vi "leitura de serial.vi"() -> ()   [LabVIEW 2025]
uses:
  <vilib>/Instr/_visa.llb/VISA Configure Serial Port (Instr).vi
panel:
  out "Waveform Chart 2":dbl(graph)
  out "output 2":dbl
  out "Waveform Chart":dbl(graph)
  out "output 1":dbl
  in  "termination char\n(0xA = '\\n' = LF)":u8=10 format="%.0x"
  out "read buffer":string
  in  "SELETOR":dbl
  out "Numeric":i32
  in  "VISA resource name":refnum<visa-resource-name>
  in  "String":string
  in  "stop":bool
  in  "baud rate (9600)":u32=9600
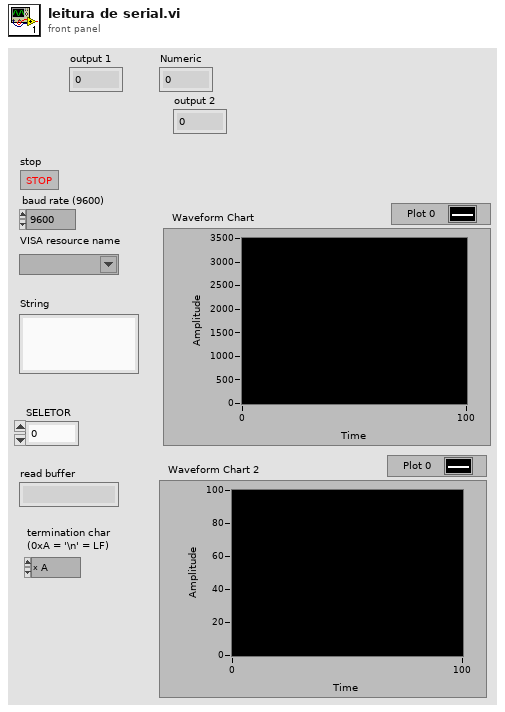
[diagram p1: front panel]
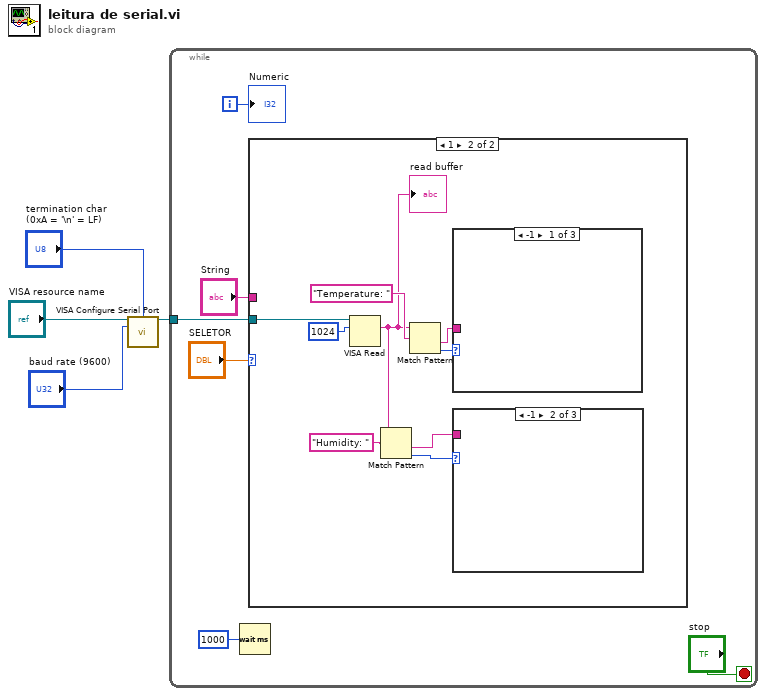
[diagram p0: block diagram]
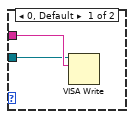
[diagram p2: hidden frame]
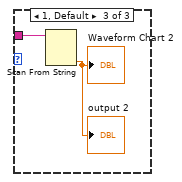
[diagram p4: hidden frame]
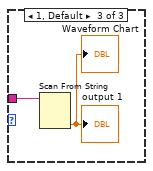
[diagram p6: hidden frame]
diagram:
  n1 = call-poly "VISA Configure Serial Port"("VISA resource name"="VISA resource name", "termination char\n(0xA = '\\n' = LF)"="termination char\n(0xA = '\\n' = LF)", "baud rate (9600)"="baud rate (9600)") -> ("VISA resource name out"=w3:refnum<visa-resource-name>)  [unwired: 11 in, 1 out]
  n2 = while {
    tunnel: w3 -> [w6]
    i -> [w8]
    stop <- "stop" stop-if-true
    n3 = Wait (ms)(milliseconds to wait=u32 1000) -> ()  [unwired: 1 out]
    n4 = case shown="1" "SELETOR" {
      tunnel: "String" -> [w12 _]
      tunnel: w6 -> [w11 w21]
      frame 0, Default {
        n5 = VISA Write(VISA resource name=w11, write buffer=w12) -> ()  [unwired: 1 in, 3 out]
      }
      frame 1 {
        n6 = VISA Read(VISA resource name=w21, byte count=1024) -> (read buffer=w17:string)  [unwired: 1 in, 3 out]
        "read buffer" <- w17
        n7 = Match Pattern(string=w17, regular expression="Humidity: ") -> (after substring=w13:string, offset past match=w14:i32)  [unwired: 1 in, 2 out]
        n8 = Match Pattern(string=w17, regular expression="Temperature: ") -> (after substring=w18:string, offset past match=w15:i32)  [unwired: 1 in, 2 out]
        n9 = case shown="-1" w15 {
          tunnel: w18 -> [_ _ w25]
          frame -1 {
          }
          frame 0 {
          }
          frame 1, Default {
            n10 = Scan From String(input string=w25) -> (output 1=→"output 1" →"Waveform Chart":dbl)  [unwired: 4 in, 3 out]
          }
        }
        n11 = case shown="-1" w14 {
          tunnel: w13 -> [_ _ w22]
          frame 0 {
          }
          frame -1 {
          }
          frame 1, Default {
            n12 = Scan From String(input string=w22) -> (output 1=→"output 2" →"Waveform Chart 2":dbl)  [unwired: 4 in, 3 out]
          }
        }
      }
    }
    "Numeric" <- w8
  }
